vi "asynchronous process.vi"(9 "Module Info In":T1, 11 "Engine Tags In":T5) -> (1 "Module Info Out":T1, 3 "Engine Tags Out":T5)   [LabVIEW 2013, in "async executor.lvlib"]
doc: "This VI exchanges data with the process method of any asynchronously running modules specified using the 'Process Method Indices' if the 'Execute?' flag for the method is TRUE. It also exchanges the data necessary for that method with the data in the main engine tags. Any errors that occur are stored to be handled at the end of the engine's execution."
uses:
  async executor/async executor.lvlib
  <vilib>/NI/Tag Bus/table/data table.ctl
  async execution info.ctl
  asynchronous process data.ctl
  async command notification.ctl
  <vilib>/NI/Tag Bus Module Framework/runtime/execution settings.ctl
  async error info.ctl
  <vilib>/NI/Tag Bus Module Framework/runtime/error classification.ctl
  Data Table with Transfer Spec.ctl
  <vilib>/NI/Tag Bus/table/transfer specification.ctl
  <vilib>/NI/Tag Bus/tag/Data Type.ctl
  Configuration/Module Decimation.ctl
  Configuration/Module Error Configuration.ctl
  Configuration/Error Actions By Category.ctl
  Configuration/Error Actions.ctl
  <vilib>/NI/Tag Bus/table/data table.lvlib
  <vilib>/NI/Tag Bus/tag/tag descriptor.lvclass
  Configuration/Standard Engine Configuration.lvclass
  <vilib>/NI/Tag Bus Module Framework/runtime/TBM module execution interface.lvclass
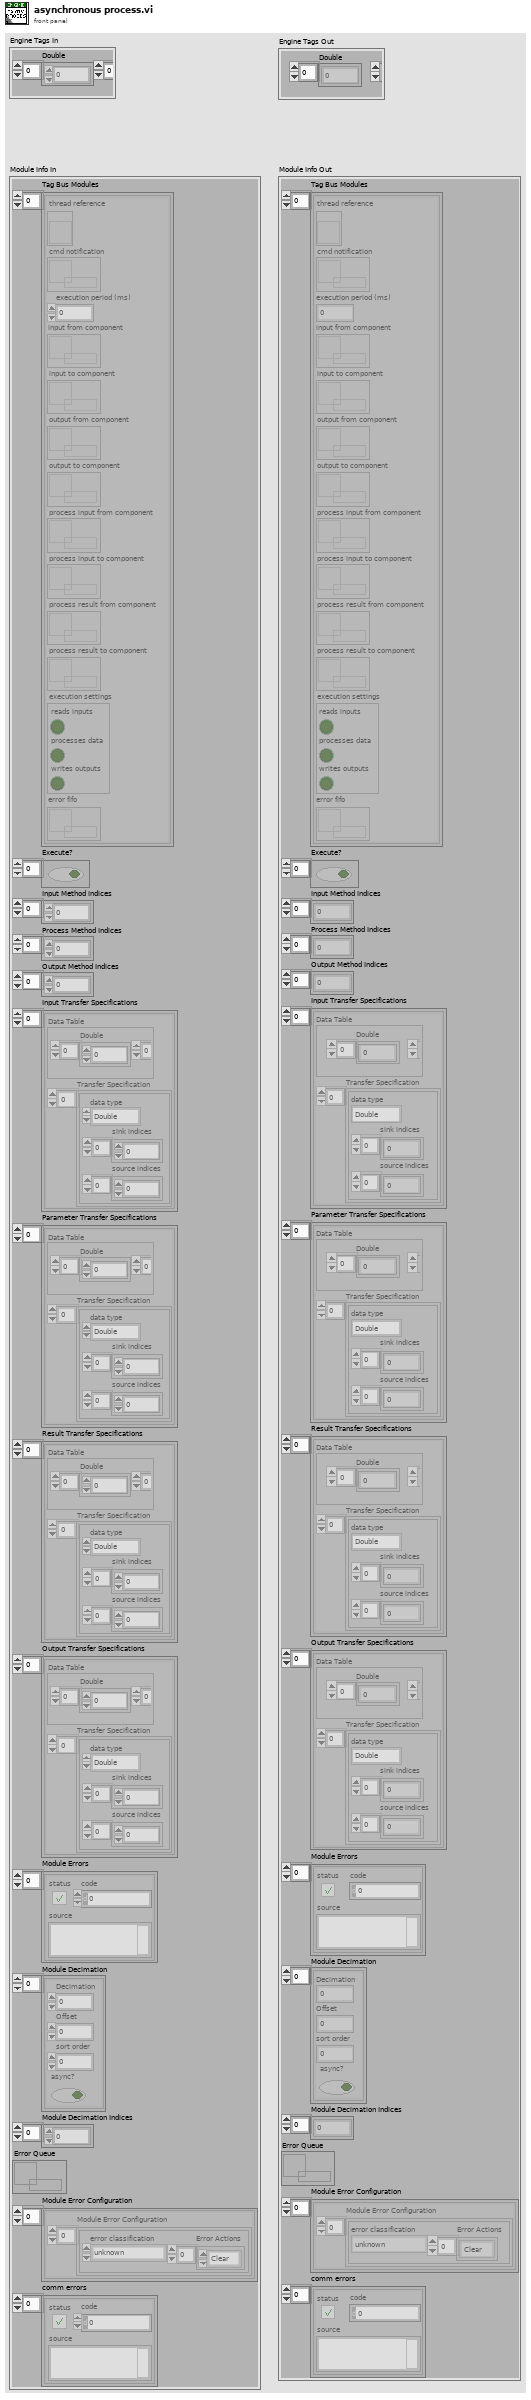
[diagram p1: front panel]
types:
  T1 = typedef "async executor.lvlib/async execution info.ctl" = cluster{"Tag Bus Modules":T2[], "Execute?":bool[], "Input Method Indices":i32[], "Process Method Indices":i32[], "Output Method Indices":i32[], "Input Transfer Specifications":T4[], "Parameter Transfer Specifications":T4[], "Result Transfer Specifications":T4[], "Output Transfer Specifications":T4[], "Module Errors":errorcluster[], "Module Decimation":T8[], "Module Decimation Indices":i32[], "Error Queue":refnum<queue>, "Module Error Configuration":T9[], "comm errors":errorcluster[]}
  T2 = typedef "async executor.lvlib/asynchronous process data.ctl" = cluster{"thread reference":refnum<vi>, "cmd notification":refnum<k33>, "execution period (ms)":i32, "input from component":refnum<queue>, "input to component":refnum<queue>, "output from component":refnum<queue>, "output to component":refnum<queue>, "process input from component":refnum<queue>, "process input to component":refnum<queue>, "process result from component":refnum<queue>, "process result to component":refnum<queue>, "execution settings":T3, "error fifo":refnum<k33>}
  T3 = typedef "TBM module execution interface.lvclass/execution settings.ctl" = cluster{"reads inputs":bool, "processes data":bool, "writes outputs":bool}
  T4 = typedef "Data Table with Transfer Spec.ctl" = cluster{"Data Table":T5, "Transfer Specification":T6[]}
  T5 = typedef "tag bus.lvlib/data table.lvlib/data table.ctl" = cluster{"Double":dbl[], "Single":sgl[], "I64":i64[], "I32":i32[], "I16":i16[], "I8":i8[], "U64":u64[], "U32":u32[], "U16":u16[], "U8":u8[], "Boolean":bool[], "String":string[], "Array of Double":cluster{"DBL Array":dbl[]}[], "Array of Single":cluster{"SGL Array":sgl[]}[], "Array of I64":cluster{"I64 Array":i64[]}[], "Array of I32":cluster{"I32 Array":i32[]}[], "Array of I16":cluster{"I16 Array":i16[]}[], "Array of I8":cluster{"I8 Array":i8[]}[], "Array of U64":cluster{"U64 Array":u64[]}[], "Array of U32":cluster{"U32 Array":u32[]}[], "Array of U16":cluster{"U16 Array":u16[]}[], "Array of U8":cluster{"U8 Array":u8[]}[], "Array of Boolean":cluster{"Boolean Array":bool[]}[], "Array of String":cluster{"String Array":string[]}[]}
  T6 = typedef "tag bus.lvlib/data table.lvlib/transfer specification.ctl" = cluster{"data type":T7, "sink indices":i32[], "source indices":i32[]}
  T7 = typedef "tag bus.lvlib/tag descriptor.lvclass/Data Type.ctl" = enum16{"Double", "Single", "I64", "I32", "I16", "I8", "U64", "U32", "U16", "U8", "Boolean", "String", "Array of Double", "Array of Single", "Array of I64", "Array of I32", "Array of I16", "Array of I8", "Array of U64", "Array of U32", "Array of U16", "Array of U8", "Array of Boolean", "Array of String"}
  T8 = typedef "Standard Engine Configuration.lvclass/Module Decimation.ctl" = cluster{"Decimation":u16, "Offset":u16, "sort order":i32, "async?":bool}
  T9 = typedef "Standard Engine Configuration.lvclass/Module Error Configuration.ctl" = cluster{"Module Error Configuration":T10[]}
  T10 = typedef "Standard Engine Configuration.lvclass/Error Actions By Category.ctl" = cluster{"error classification":T11, "Error Actions":T12[]}
  T11 = typedef "TBM module execution interface.lvclass/error classification.ctl" = enum16{"unknown", "none", "trivial", "recoverable", "critical"}
  T12 = typedef "Standard Engine Configuration.lvclass/Error Actions.ctl" = enum16{"Clear", "Notify", "Stop Component", "Stop Engine", "Safe State", "Attempt Recovery"}
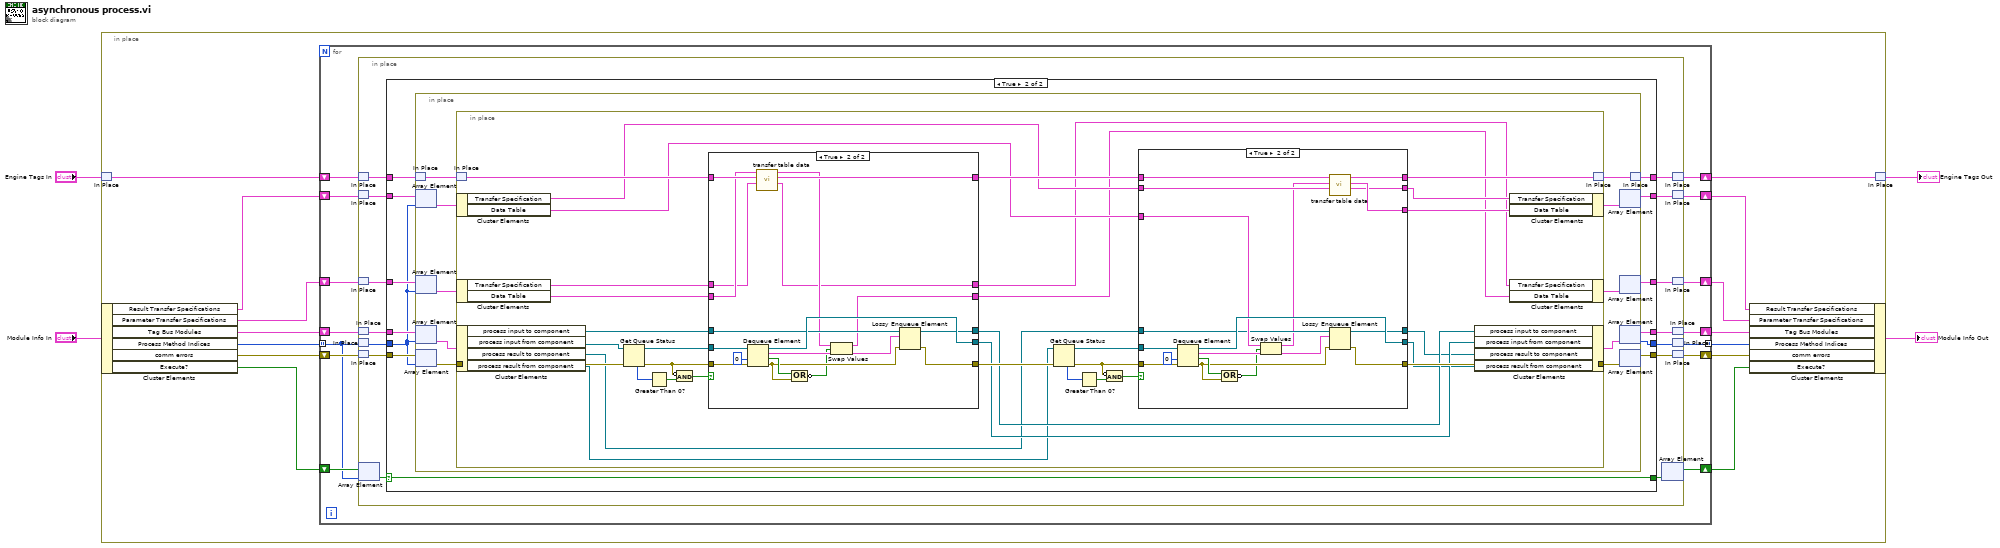
[diagram p0: block diagram]
diagram:
  n1 = in-place {
    n2 = in-place-match #1("Engine Tags In") -> (w17:T5)
    n3 = in-place-cluster #2("Module Info In") -> ("Result Transfer Specifications"=w6:T4[], "Parameter Transfer Specifications"=w15:T4[], "Tag Bus Modules"=w12:T2[], "Process Method Indices"=w18:i32[], "comm errors"=w14:errorcluster[], "Execute?"=w8:bool[])
    n4 = for {
      shift-right: [w25] -> w11
      shift-left: w12 -> [w26]
      tunnel: w18 -> [w22] mode=indexing
      shift-right: [w29] -> w16
      shift-left: w17 -> [w30]
      shift-right: [w27] -> w13
      shift-left: w15 -> [w28]
      shift-right: [w23] -> w10
      shift-left: w14 -> [w24]
      tunnel: [w21] -> w9 mode=indexing
      shift-right: [w31] -> w7
      shift-left: w8 -> [w32]
      shift-right: [w19] -> w5
      shift-left: w6 -> [w20]
      n5 = in-place {
        n6 = in-place-match #3(w30) -> (w44:T5)
        n7 = in-place-match #4(w20) -> (w33:T4[])
        n8 = in-place-match #5(w28) -> (w42:T4[])
        n9 = in-place-match #6(w26) -> (w40:T2[])
        n10 = in-place-match #7(w22) -> (w36:i32)
        n11 = in-place-match #8(w24) -> (w38:errorcluster[])
        n12 = in-place-array #9(w32, w22) -> (w46:bool)
        n13 = case shown="True" w46 {
          selector: w46 -> [w48 w57]
          tunnel: w44 -> [w53 w66]
          tunnel: [w53 w65] -> w43
          tunnel: w42 -> [w52 w64]
          tunnel: w40 -> [w51 w63]
          tunnel: w38 -> [w49 w62]
          tunnel: [w52 w61] -> w41
          tunnel: [w49 w60] -> w37
          tunnel: [w51 w59] -> w39
          tunnel: w36 -> [w50 w54]
          tunnel: [w50 w58] -> w35
          tunnel: [w48 w57] -> w45
          tunnel: [w47 w55] -> w34
          tunnel: w33 -> [w47 w56]
          frame False {
          }
          frame True {
            n14 = in-place {
              n15 = in-place-match #10(w66) -> (w76:T5)
              n16 = in-place-array #11(w56, w54) -> (w68:T4)
              n17 = in-place-array #12(w64, w54) -> (w74:T4)
              n18 = in-place-array #13(w63, w54) -> (w72:T2)
              n19 = in-place-array #14(w62, w54) -> (w70:errorcluster)
              n20 = in-place {
                in-place-border: w70 -> [w106]
                in-place-border: [w84] -> w69
                n21 = in-place-match #15(w76) -> (w108:T5)
                n22 = in-place-cluster #16(w68) -> ("Transfer Specification"=w89:T6[], "Data Table"=w86:T5)
                n23 = in-place-cluster #17(w74) -> ("Transfer Specification"=w107:T6[], "Data Table"=w105:T5)
                n24 = in-place-cluster #18(w72) -> ("process input to component"=w104:refnum<queue>, "process input from component"=w103:refnum<queue>, "process result to component"=w77:refnum<queue>, "process result from component"=w78:refnum<queue>)
                n25 = Get Queue Status(queue=w103, error in (no error)=w106) -> (queue out=w102:refnum<queue>, error out=w98:errorcluster, # elements in queue=w101:i32)  [unwired: 1 in, 5 out]
                n26 = Greater Than 0?(x=w101) -> (x > 0?=w100:bool)
                n27 = Compound Arithmetic op=AND(invert w98, w100) -> (w99:bool)
                n28 = case shown="True" w99 {
                  tunnel: w108 -> [w134 w145]
                  tunnel: [w134 w144] -> w91
                  tunnel: [w136 w148] -> w83
                  tunnel: w107 -> [w135 w141]
                  tunnel: [w135 w140] -> w85
                  tunnel: [w139 w156] -> w81
                  tunnel: w105 -> [w136 w143]
                  tunnel: w104 -> [w138 w153]
                  tunnel: [w138 w152] -> w82
                  tunnel: [w137 w151] -> w92
                  tunnel: w102 -> [w139 w150]
                  tunnel: w98 -> [w137 w149]
                  frame False {
                  }
                  frame True {
                    n29 = Dequeue Element(queue=w150, timeout in ms (-1)=0, error in (no error)=w149) -> (queue out=w156:refnum<queue>, element=w154:T5, timed out?=w157:bool, error out=w155:errorcluster)
                    n30 = call <vilib>:"transfer table data.vi"("transfer specification in"=w141, "data table source in"=w145, "data table sink in"=w143) -> ("transfer specification out"=w140:T6[], "data table source out"=w144:T5, "data table sink out"=w142:T5)  [unwired: 6 in]
                    n31 = Compound Arithmetic op=OR(w157, w155) -> (invert w146:bool)
                    n32 = Swap Values(12:w142, 13:w146, 14:w154) -> (1:w148:T5, 3:w147:T5)
                    n33 = Lossy Enqueue Element(queue=w153, element=w147, error in (no error)=w155) -> (queue out=w152:refnum<queue>, error out=w151:errorcluster)  [unwired: 2 out]
                  }
                }
                n34 = Get Queue Status(queue=w78, error in (no error)=w92) -> (queue out=w97:refnum<queue>, error out=w93:errorcluster, # elements in queue=w96:i32)  [unwired: 1 in, 5 out]
                n35 = Greater Than 0?(x=w96) -> (x > 0?=w95:bool)
                n36 = Compound Arithmetic op=AND(invert w93, w95) -> (w94:bool)
                n37 = case shown="True" w94 {
                  tunnel: w91 -> [w109 w133]
                  tunnel: [w109 w132] -> w90
                  tunnel: [w111 w131] -> w87
                  tunnel: w89 -> [w110 w130]
                  tunnel: [w110 w129] -> w88
                  tunnel: [w114 w126] -> w80
                  tunnel: w86 -> [w111 w123]
                  tunnel: w77 -> [w113 w122]
                  tunnel: [w113 w121] -> w79
                  tunnel: [w112 w120] -> w84
                  tunnel: w97 -> [w114 w119]
                  tunnel: w93 -> [w112 w118]
                  frame False {
                  }
                  frame True {
                    n38 = Dequeue Element(queue=w119, timeout in ms (-1)=0, error in (no error)=w118) -> (queue out=w126:refnum<queue>, element=w124:T5, timed out?=w127:bool, error out=w125:errorcluster)
                    n39 = Compound Arithmetic op=OR(w127, w125) -> (invert w115:bool)
                    n40 = Swap Values(12:w123, 13:w115, 14:w124) -> (1:w117:T5, 3:w116:T5)
                    n41 = call <vilib>:"transfer table data.vi"("transfer specification in"=w130, "data table source in"=w117, "data table sink in"=w133) -> ("transfer specification out"=w129:T6[], "data table source out"=w131:T5, "data table sink out"=w132:T5)  [unwired: 6 in]
                    n42 = Lossy Enqueue Element(queue=w122, element=w116, error in (no error)=w125) -> (queue out=w121:refnum<queue>, error out=w120:errorcluster)  [unwired: 2 out]
                  }
                }
                n43 = in-place-cluster #18("process input to component"=w82, "process input from component"=w81, "process result to component"=w79, "process result from component"=w80) -> (w71:T2)
                n44 = in-place-cluster #16("Transfer Specification"=w88, "Data Table"=w87) -> (w67:T4)
                n45 = in-place-cluster #17("Transfer Specification"=w85, "Data Table"=w83) -> (w73:T4)
                n46 = in-place-match #15(w90) -> (w75:T5)
              }
              n47 = in-place-array #11(w67) -> (w55:T4[])  [unwired: 1 out]
              n48 = in-place-array #12(w73) -> (w61:T4[])  [unwired: 1 out]
              n49 = in-place-array #13(w71) -> (w59:T2[], w58:i32)
              n50 = in-place-array #14(w69) -> (w60:errorcluster[])  [unwired: 1 out]
              n51 = in-place-match #10(w75) -> (w65:T5)
            }
          }
        }
        n52 = in-place-array #9(w45) -> (w31:bool[])  [unwired: 1 out]
        n53 = in-place-match #3(w43) -> (w29:T5)
        n54 = in-place-match #4(w34) -> (w19:T4[])
        n55 = in-place-match #5(w41) -> (w27:T4[])
        n56 = in-place-match #6(w39) -> (w25:T2[])
        n57 = in-place-match #7(w35) -> (w21:i32)
        n58 = in-place-match #8(w37) -> (w23:errorcluster[])
      }
    }
    n59 = in-place-cluster #2("Result Transfer Specifications"=w5, "Parameter Transfer Specifications"=w13, "Tag Bus Modules"=w11, "Process Method Indices"=w9, "comm errors"=w10, "Execute?"=w7) -> (→"Module Info Out":T1)
    n60 = in-place-match #1(w16) -> (→"Engine Tags Out":T5)
  }
